vi "Start Module.vi"(6 "Show Main VI Diagram on Init (F)":bool, 8 "error in":errorcluster, 11 "Run as Singleton? (F)":bool) -> (0 "error out":errorcluster, 1 "Wait for Event Sync?":bool, 2 "My Cloneable Module Broadcast Events":T1, 3 "Module ID":i32)   [LabVIEW 2022 SP3, in "My Cloneable Module.lvlib"]
doc: "Launches an instance of the module Main VI. After calling this VI, you can optionally register for broadcast events from the module by wiring the broadcast events output of this VI to a <b>Register For Events</b> function. \n\nAfter the optional Register For Events function call, you should always call the <b>Synchronize Module Events.vi</b> for this module with the 'Wait for Event Sync?' output of this VI to the corresponding input of the Synchronize Module Events.vi. \n\nTo see an example of the proper wiring pattern, see the \"Run New Module: Value Change\" event frame in the API Tester VI for this module.\n_____\nBased on DQMH Project Template 7.0.1.1316."
uses:
  My Cloneable Module.lvlib
  Broadcast Events--cluster.ctl
  Did Init Argument--cluster.ctl
  Status Updated Argument--cluster.ctl
  Error Reported Argument--cluster.ctl
  Do Something Argument--cluster.ctl
  Stop Argument--cluster.ctl
  Get Module Execution Status Argument--cluster.ctl
  Module Running State--enum.ctl
  <vilib>/Delacor/Delacor QMH/Libraries/Cloneable Module Admin_class/Delacor_lib_QMH_Cloneable Module Admin.lvclass
  C:/Program Files (x86)/National Instruments/LabVIEW 2022/vi.lib/Delacor/Delacor QMH/Libraries/Module Admin_class/Delacor_lib_QMH_Module Admin.lvclass
  VI Reference Management/Main VI Type--strict_vi_ref.ctl
  <vilib>/Delacor/Delacor QMH/Libraries/Cloneable Module Admin_class/Delacor_lib_QMH_Cloneable Module Admin.lvclass/Delacor_lib_QMH_Cloneable Module Admin.ctl
  <vilib>/Delacor/Delacor QMH/Libraries/Module Admin_class/Delacor_lib_QMH_Module Admin.lvclass/Delacor_lib_QMH_Module Admin.ctl
  <vilib>/Delacor/Delacor QMH/Libraries/Cloneable Module Admin_class/Delacor_lib_QMH_Set Module ID.vi
  <vilib>/Delacor/Delacor QMH/Libraries/Module Admin_class/Delacor_lib_QMH_Set External Launch.vi
  Main.vi
  Clone Registration/Clone Registration.lvlib
  VI Reference Management/VI Reference Management.lvlib
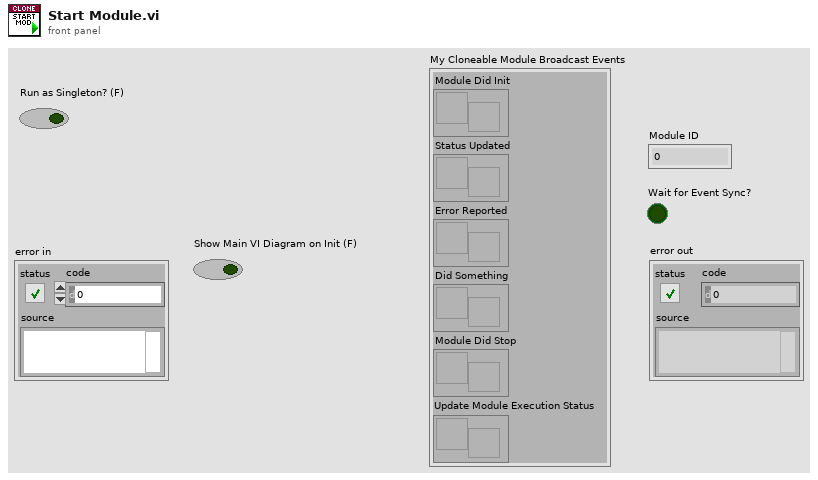
[diagram p1: front panel]
types:
  T1 = typedef "My Cloneable Module.lvlib/Broadcast Events--cluster.ctl" = cluster{"Module Did Init":refnum<user-event>, "Status Updated":refnum<user-event>, "Error Reported":refnum<user-event>, "Did Something":refnum<user-event>, "Module Did Stop":refnum<user-event>, "Update Module Execution Status":refnum<user-event>}
  T2 = typedef "My Cloneable Module.lvlib/Module Running State--enum.ctl" = enum16{"Not Running", "Running as Cloneable", "Running as Singleton"}
  T3 = enum32{"Bad", "Idle", "Run top level", "Running"}
  T4 = typedef "My Cloneable Module.lvlib/VI Reference Management.lvlib/Main VI Type--strict_vi_ref.ctl" = refnum<vi>
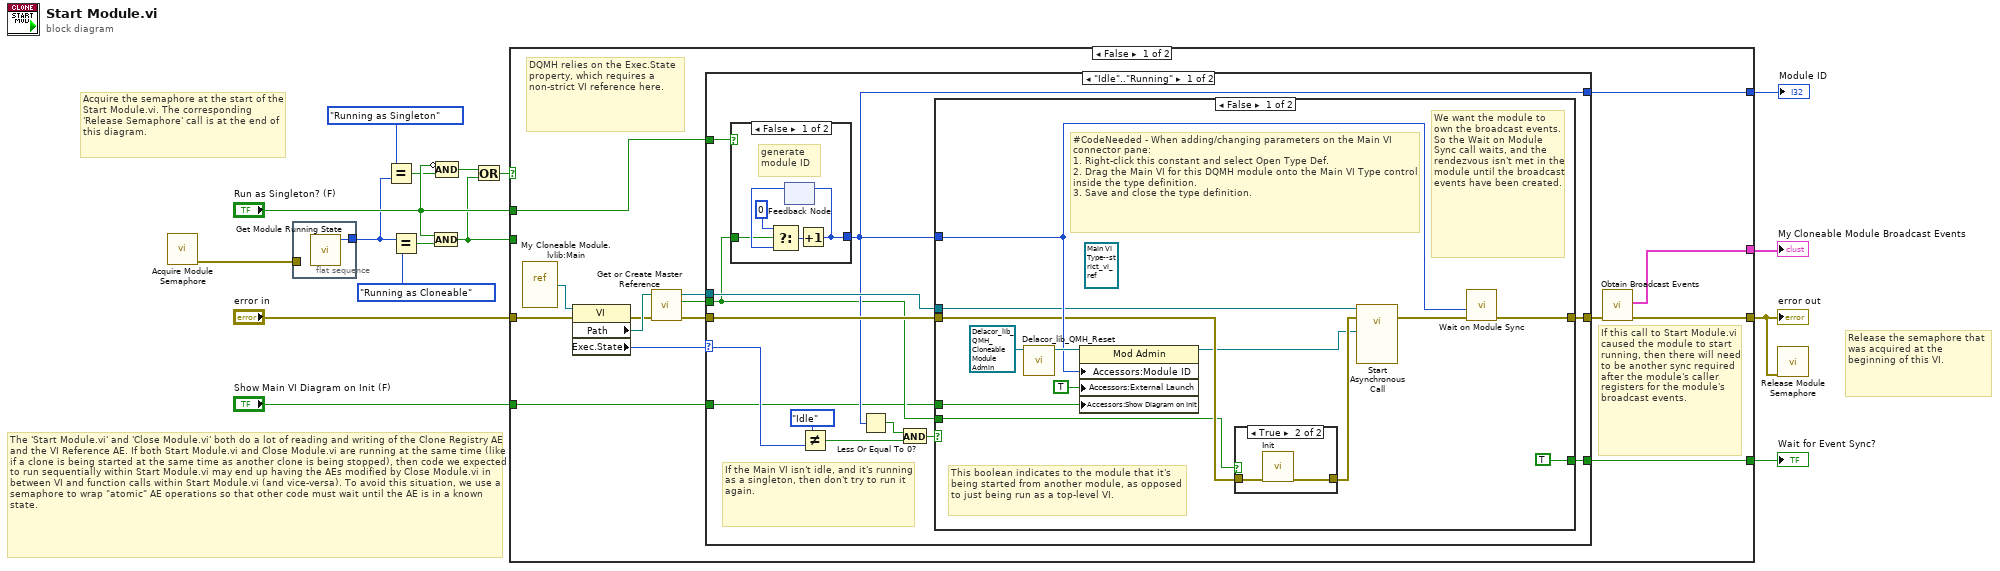
[diagram p0: block diagram]
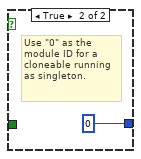
[diagram p2: hidden frame]
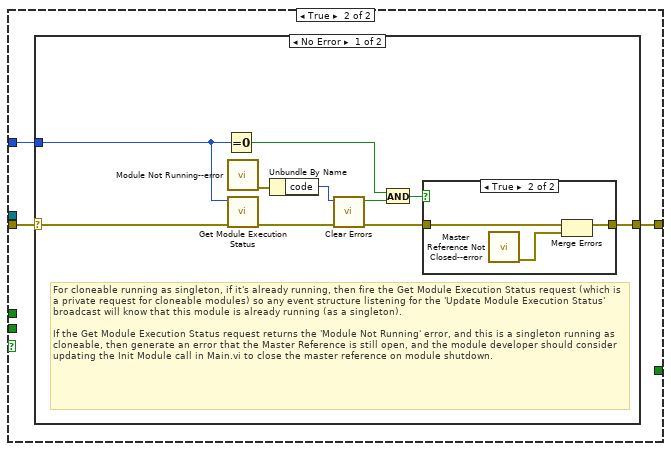
[diagram p4: hidden frame]
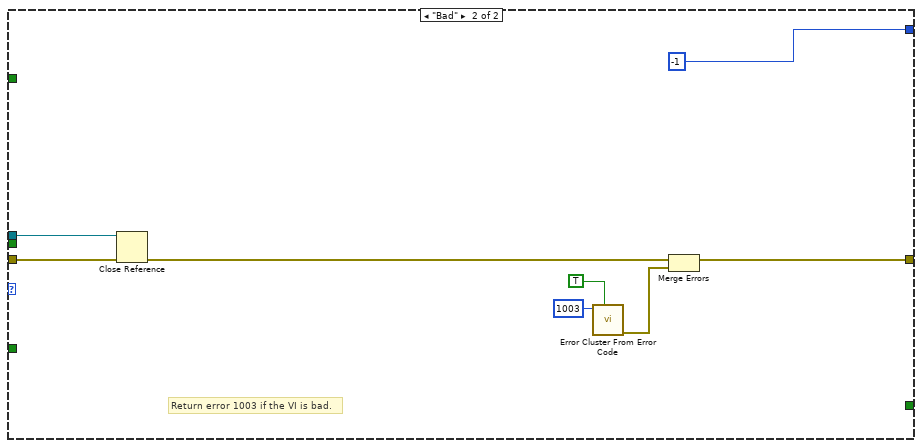
[diagram p7: hidden frame]
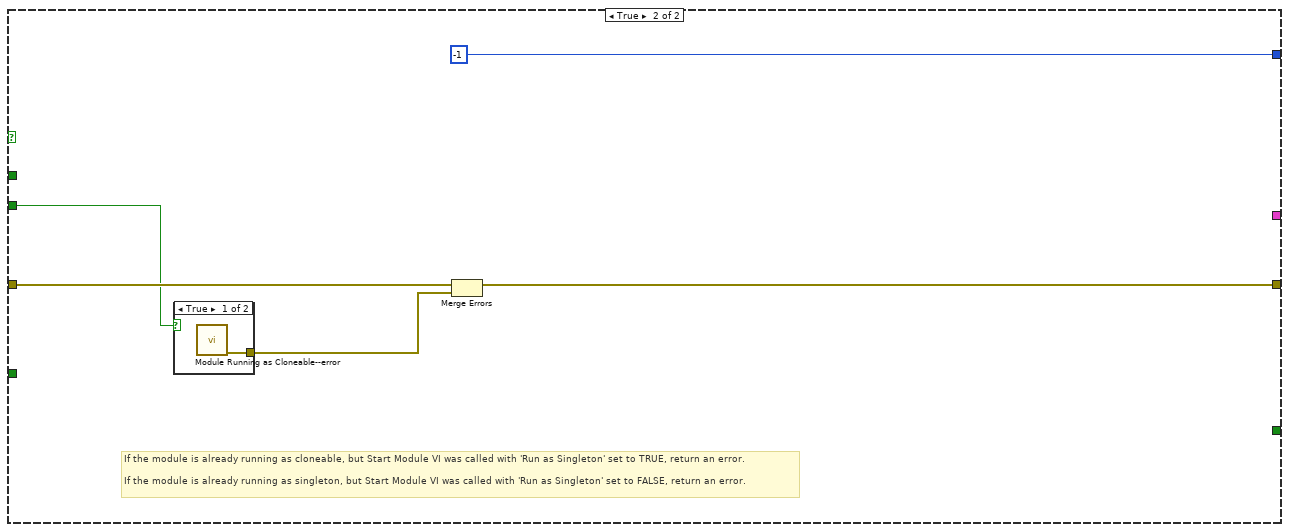
[diagram p8: hidden frame]
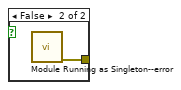
[diagram p9: hidden frame]
diagram:
  # "Release the semaphore that was acquired at the beginning of this VI."
  # "The 'Start Module.vi' and 'Close Module.vi' both do a lot of reading and writing of the Clone Registry AE and the VI Reference AE. If both Start Module.vi and Close Module.vi are running at the same time (like if a clone is being started at the same time as another clone is being stopped), then code we expected to run sequentially within Start Module.vi may end up having the AEs modified by Close Module.vi in between VI and function calls within Start Module.vi (and vice-versa). To avoid this situation, we use a semaphore to wrap \"atomic\" AE operations so that other code must wait until the AE is in a known state."
  # "Acquire the semaphore at the start of the Start Module.vi. The corresponding 'Release Semaphore' call is at the end of this diagram."
  n1 = call "Acquire Module Semaphore.vi"() -> ("error out"=w3:errorcluster)  [unwired: 11 in]
  n2 = flat-sequence {
    tunnel: [w17] -> w6
    tunnel: w3 -> [_]
    frame #0 {
      n3 = call "Get Module Running State.vi"() -> ("Module Running State"=w17:T2)  [unwired: 11 in]
    }
  }
  n4 = Equal?(x=Module_Running_State--enum."Running as Singleton", y=w6) -> (x = y?=w7:bool)
  n5 = Equal?(x=w6, y=Module_Running_State--enum."Running as Cloneable") -> (x = y?=w11:bool)
  n6 = And(x="Run as Singleton? (F)", y=w11) -> (x .and. y?=w4:bool)
  n7 = Compound Arithmetic op=AND(invert "Run as Singleton? (F)", w7) -> (w9:bool)
  n8 = Or(x=w9, y=w4) -> (x .or. y?=w10:bool)
  n9 = case shown="False" w10 {
    tunnel: "error in" -> [w32 w98]
    tunnel: [w30 w97] -> w2
    tunnel: [w29 _] -> w15
    tunnel: [w28 _] -> w14
    tunnel: [w24 -1] -> w13
    tunnel: "Run as Singleton? (F)" -> [w20 _]
    tunnel: w4 -> [_ w94]
    tunnel: "Show Main VI Diagram on Init (F)" -> [w18 _]
    frame False {
      # "DQMH relies on the Exec.State property, which requires a non-strict VI reference here."
      # "If this call to Start Module.vi caused the module to start running, then there will need to be another sync required after the module's caller registers for the module's broadcast events."
      n10 = vi-ref "My Cloneable Module.lvlib:Main.vi"() -> (w23:refnum<vi>)
      n11 = property class="VI"(reference=w23, error in=w32) -> (error out=w26:errorcluster, "Path"=w27:path, "Exec.State"=w21:T3)  [unwired: 1 out]
      n12 = call "Get or Create Master Reference.vi"("error in"=w26, "Main VI Path"=w27) -> ("error out"=w25:errorcluster, "New Reference Created"=w19:bool, "Master Reference"=w22:T4)  [unwired: 7 in]
      n13 = case shown="\"Idle\"..\"Running\"" w21 {
        selector: w21 -> [w41 _]
        tunnel: w25 -> [w45 w93]
        tunnel: w22 -> [w43 w92]
        tunnel: [w42 w90] -> w31
        tunnel: [w44 _] -> w28
        tunnel: [w36 -1] -> w24
        tunnel: w20 -> [w35 _]
        tunnel: w19 -> [w34 _]
        tunnel: w18 -> [w33 _]
        frame "Idle".."Running" {
          # "If the Main VI isn't idle, and it's running as a singleton, then don't try to run it again."
          n14 = case shown="False" w35 {
            tunnel: [w50 0] -> w36
            tunnel: w34 -> [w46 _]
            frame False {
              # "generate module ID"
              n15 = feedback #1() -> (w48:i32)  [unwired: 1 in]
              n16 = Select(t=0, s=w46, f=w48) -> (s? t:f=w49:i32)
              n17 = Increment(x=w49) -> (x+1=w50:i32)
              n18 = feedback-in #1(w50) -> ()
            }
            frame True {
              # "Use \"0\" as the module ID for a cloneable running as singleton."
            }
          }
          n19 = Not Equal?(x=T3."Idle", y=w41) -> (x != y?=w39:bool)
          n20 = Less Or Equal To 0?(x=w36) -> (x <= 0?=w37:bool)
          n21 = And(x=w37, y=w39) -> (x .and. y?=w38:bool)
          n22 = case shown="False" w38 {
            tunnel: w45 -> [w56 w69]
            tunnel: [TRUE _] -> w44
            tunnel: w43 -> [w55 _]
            tunnel: [w59 w68] -> w42
            tunnel: w36 -> [w60 w70]
            tunnel: w34 -> [w53 _]
            tunnel: w33 -> [w52 _]
            frame False {
              (unwired) T4 refnum ("Main VI Type")
              # "#CodeNeeded - When adding/changing parameters on the Main VI connector pane:\n1. Right-click this constant and select Open Type Def.\n2. Drag the Main VI for this DQMH module onto the Main VI Type control inside the type definition.\n3. Save and close the type definition."
              # "We want the module to own the broadcast events. So the Wait on Module Sync call waits, and the rendezvous isn't met in the module until the broadcast events have been created."
              # "This boolean indicates to the module that it's being started from another module, as opposed to just being run as a top-level VI."
              n23 = call-dynamic "Delacor_lib_QMH_Reset.vi"("Mod Admin in"=refnum<class "Delacor_lib_QMH_Cloneable Module Admin.lvclass"> refnum) -> ("Mod Admin out"=w63:refnum<class "Delacor_lib_QMH_Cloneable Module Admin.lvclass">)  [unwired: 9 in, 1 out]
              n24 = property class="Mod Admin"(reference=w63, "Accessors:Module ID"=w60, "Accessors:External Launch"=TRUE, "Accessors:Show Diagram on Init"=w52) -> (reference out=w54:refnum<class "Delacor_lib_QMH_Cloneable Module Admin.lvclass">)  [unwired: 1 in, 1 out]
              n25 = case shown="True" w53 {
                tunnel: [w65 w67] -> w57
                tunnel: w56 -> [w65 w66]
                frame False {
                }
                frame True {
                  n26 = call "Init.vi"("error in"=w66) -> ("error out"=w67:errorcluster)  [unwired: 7 in, 3 out]
                }
              }
              n27 = call-by-ref "Start Asynchronous Call"(reference=w55, error in=w57, "Module Admin"=w54) -> (error out=w58:errorcluster)  [unwired: 11 in, 1 out]
              n28 = call "Wait on Module Sync.vi"("error in"=w58, "Module ID"=w60) -> ("error out"=w59:errorcluster)  [unwired: 9 in]
            }
            frame True {
              n29 = case shown="No Error" w69 {
                selector: w69 -> [w80 w85]
                tunnel: w70 -> [w78 _]
                tunnel: [w71 w85] -> w68
                frame No Error {
                  # "For cloneable running as singleton, if it's already running, then fire the Get Module Execution Status request (which is a private request for cloneable modules) so any event structure listening for the 'Update Module Execution Status' broadcast will know that this module is already running (as a singleton).\n\nIf the Get Module Execution Status request returns the 'Module Not Running' error, and this is a singleton running as cloneable, then generate an error that the Master Reference is still open, and the module developer should consider updating the Init Module call in Main.vi to close the master reference on module shutdown."
                  n30 = Equal To 0?(x=w78) -> (x = 0?=w74:bool)
                  n31 = call "Module Not Running--error.vi"() -> ("error out"=w77:errorcluster)  [unwired: 11 in]
                  n32 = call "Get Module Execution Status.vi"("error in"=w80, "Module ID"=w78) -> ("error out"=w79:errorcluster)  [unwired: 9 in]
                  n33 = Unbundle By Name(w77) -> ("code"=w76:i32)
                  n34 = call <vilib>:"Clear Errors.vi"("error in (no error)"=w79, "specific error code to clear (0: all)"=w76) -> ("error out"=w73:errorcluster, "specific error cleared?"=w75:bool)  [unwired: 4 in]
                  n35 = And(x=w74, y=w75) -> (x .and. y?=w72:bool)
                  n36 = case shown="True" w72 {
                    tunnel: w73 -> [w81 w84]
                    tunnel: [w81 w82] -> w71
                    frame False {
                    }
                    frame True {
                      n37 = call "Master Reference Not Closed--error.vi"() -> ("error out"=w83:errorcluster)  [unwired: 11 in]
                      n38 = Merge Errors(w84, w83) -> (w82:errorcluster)
                    }
                  }
                }
                frame Error {
                }
              }
            }
          }
        }
        frame "Bad" {
          # "Return error 1003 if the VI is bad."
          n39 = Close Reference(reference=w92, error in (no error)=w93) -> (error out=w91:errorcluster)
          n40 = call <vilib>:"Error Cluster From Error Code.vi"("show call chain? (False)"=TRUE, "error code (0)"=1003) -> ("error out"=w88:errorcluster)  [unwired: 7 in]
          n41 = Merge Errors(w91, w88) -> (w90:errorcluster)
        }
      }
      n42 = call "Obtain Broadcast Events.vi"("error in"=w31) -> ("error out"=w30:errorcluster, "My Cloneable Module Broadcast Events"=w29:T1)  [unwired: 9 in]
    }
    frame True {
      # "If the module is already running as cloneable, but Start Module VI was called with 'Run as Singleton' set to TRUE, return an error.\n\nIf the module is already running as singleton, but Start Module VI was called with 'Run as Singleton' set to FALSE, return an error."
      n43 = case shown="True" w94 {
        tunnel: [w99 w100] -> w95
        frame True {
          n44 = call "Module Running as Cloneable--error.vi"() -> ("error out"=w99:errorcluster)  [unwired: 11 in]
        }
        frame False {
          n45 = call "Module Running as Singleton--error.vi"() -> ("error out"=w100:errorcluster)  [unwired: 11 in]
        }
      }
      n46 = Merge Errors(w98, w95) -> (w97:errorcluster)
    }
  }
  "error out" <- w2
  "My Cloneable Module Broadcast Events" <- w15
  "Wait for Event Sync?" <- w14
  "Module ID" <- w13
  n47 = call "Release Module Semaphore.vi"("error in"=w2) -> ()  [unwired: 10 in, 1 out]
